vi "Read Transfer Buffer.vi"(8 "error in (no error)":errorcluster, 10 "Transfer":refnum<class "Transfer.lvclass">, 11 "UDPlog Transceiver in":refnum<class "UDPlog Transceiver.lvclass">) -> (0 "error out":errorcluster, 1 "data":string, 3 "UDPlog Transceiver out":refnum<class "UDPlog Transceiver.lvclass">)   [LabVIEW 2023, in "UDPlog.lvlib" / "UDPlog Transceiver.lvclass"]
uses:
  UDPlog Transceiver.lvclass
  UDPlog Transceiver.lvclass/UDPlog Transceiver.ctl
  <vilib>/AddOns/VeriStand Custom Device Scripting APIs/Data Sharing Framework/DSF Core.lvlibp/Classes/Transfer/Transfer.lvclass
  <vilib>/AddOns/VeriStand Custom Device Scripting APIs/Data Sharing Framework/DSF Core.lvlibp/Classes/Buffer/Buffer.lvclass
  <vilib>/AddOns/VeriStand Custom Device Scripting APIs/Data Sharing Framework/DSF Core.lvlibp/Classes/Buffer/Read Buffer 1D U8.vi
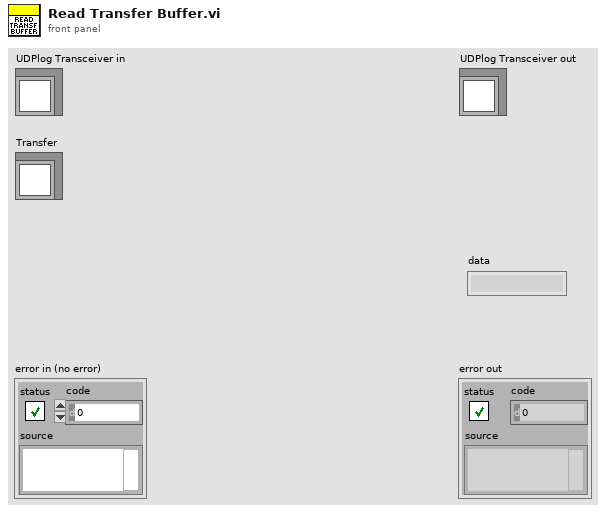
[diagram p1: front panel]
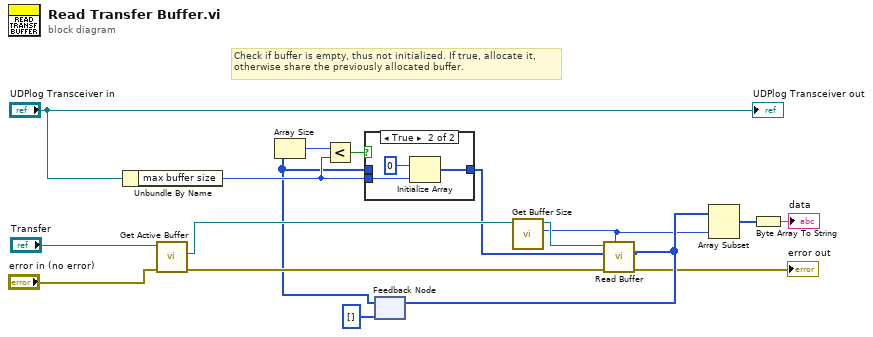
[diagram p0: block diagram]
diagram:
  # "Check if buffer is empty, thus not initialized. If true, allocate it,\notherwise share the previously allocated buffer."
  n1 = Unbundle By Name("UDPlog Transceiver in") -> ("max buffer size"=w11:u64)
  n2 = call <vilib>:"Get Active Buffer.vi"("error in (no error)"="error in (no error)", "Transfer in"="Transfer") -> ("error out"=w7:errorcluster, "Buffer"=w10:refnum<class "Buffer.lvclass">)  [unwired: 7 in, 1 out]
  n3 = feedback #1(u8[] []) -> (w6:u8[])
  n4 = Array Size(array=w6) -> (size(s)=w13:i32)
  n5 = Less?(x=w13, y=w11) -> (x < y?=w14:bool)
  n6 = case shown="True" w14 {
    tunnel: w6 -> [w18 _]
    tunnel: [w18 w21] -> w8
    tunnel: w11 -> [_ w19]
    frame False {
    }
    frame True {
      n7 = Initialize Array(u8 0 ("Numeric"), w19) -> (w21:u8[])
    }
  }
  n8 = call <vilib>:"Get Buffer Size.vi"("Buffer in"=w10) -> ("buffer size"=w3:u64, "Buffer out"=w9:refnum<class "Buffer.lvclass">)  [unwired: 9 in]
  n9 = call-poly <vilib>:"Read Buffer.vi"("count (-1: rest)"=w3, "error in (no error)"=w7, "dst array in"=w8, "Buffer in"=w9) -> ("error out"=→"error out":errorcluster, "dst array out"=w4:u8[])  [unwired: 4 in, 2 out]
  n10 = feedback-in #1(w4) -> ()
  n11 = Array Subset(array=w4, length=w3) -> (w5:u8[])  [unwired: 1 in]
  n12 = Byte Array To String(unsigned byte array=w5) -> (string=→"data":string)
  "UDPlog Transceiver out" <- "UDPlog Transceiver in"
